vi "Read Waveform.vi"(0 "VISA resource name":refnum<visa-resource-name>, 5 "Trace Number (0: Scope Trace or Record)":i32(ring) items=["Scope Trace or Record", "Trend Plot", "Persistence", "Reference Trace", "Spectrum"], 7 "Channel (1: Channel A)":i32(ring)=1 items=["Channel A"=1, "Channel B"=2, "Channel C"=5, "Channel D"=6], 11 "error in (no error)":errorcluster) -> (3 "Y Unit":string, 4 "VISA resource name out":refnum<visa-resource-name>, 6 "Waveform":cluster{dbl[], "Max Data":dbl[]}[](graph), 8 "Overload":dbl format="%#_4e", 10 "Underload":dbl format="%#_4e", 14 "X Unit":string, 15 "error out":errorcluster)   [LabVIEW 2014, in "Fluke 190 Series II.lvlib"]
doc: "Reads and returns the trace data of a waveform from the Scopemeter."
uses:
  Fluke 190 Series II.lvlib
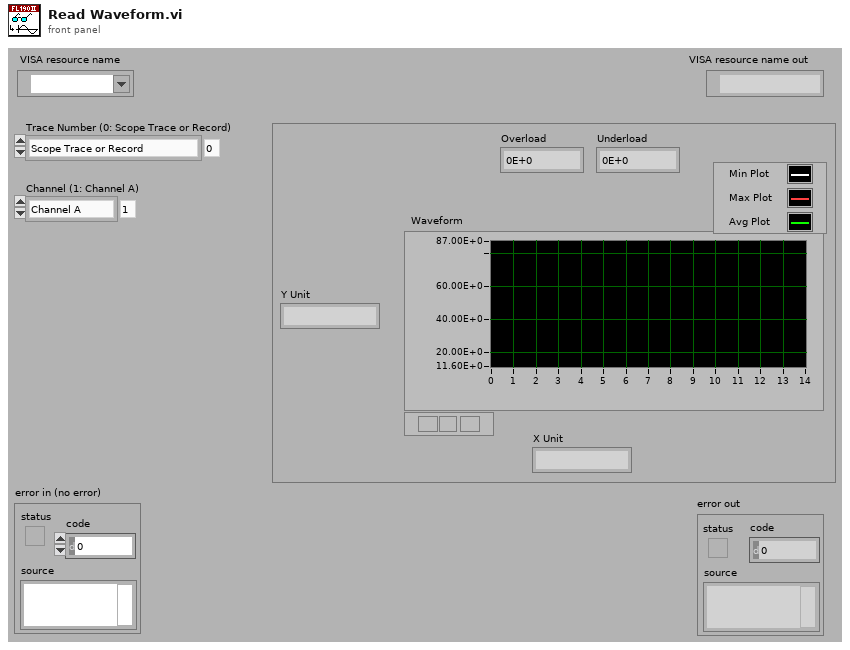
[diagram p1: front panel]
types:
  T1 = cluster{"Trace Result":u8, "Y Unit":u8, "X Unit ":u8, "Y Divisions":u16, "X Divisions":u16, "Y Scale":dbl, "X Scale":dbl, "Y Step":u8, "X Step":u8, "Y Offset":dbl, "X Offset":dbl, "Y Resolution":dbl, "X Resolution":dbl, "Y at 0":dbl, "X at 0":dbl, "Date Stamp":string, "Time Stamp":string}
  T2 = cluster{"Sample Format":i16, "Sample Pairing":u8, "Sample Byte Size":u8, "Overload":dbl, "Underload":dbl, "Invalid Samples":dbl, "Number of Samples":u16}
  T3 = cluster{"Min Data":dbl[], "Max Data":dbl[], "Avg Data":dbl[]}
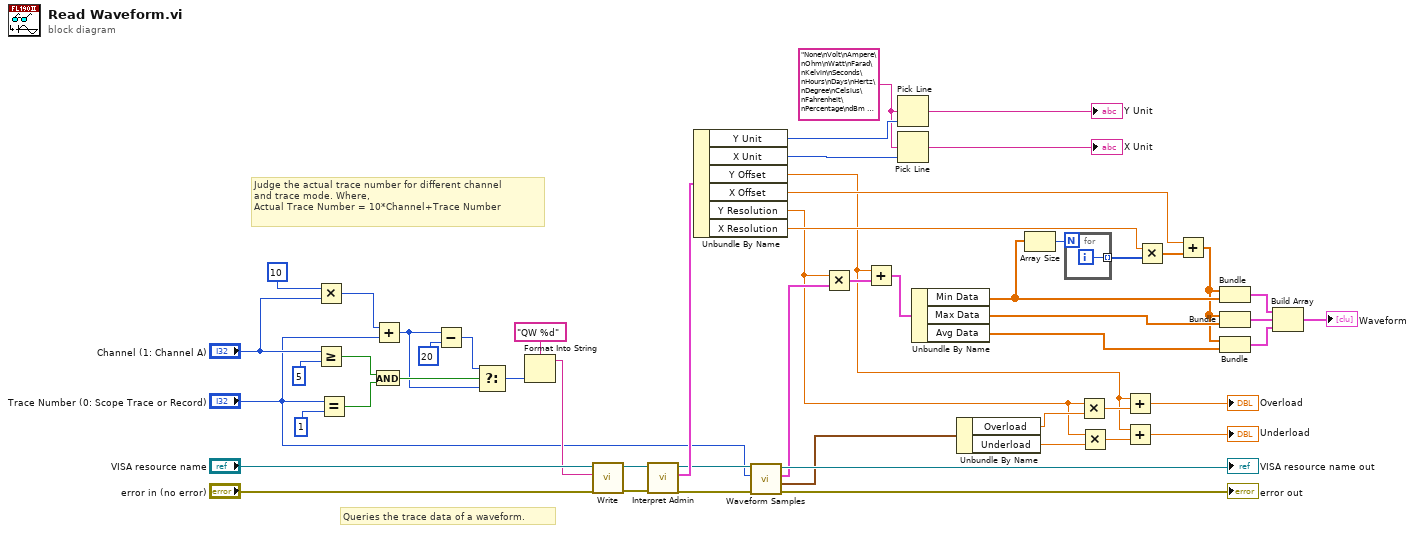
[diagram p0: block diagram]
diagram:
  w35 = "None\nVolt\nAmpere\nOhm\nWatt\nFarad\nKelvin\nSeconds\nHours\nDays\nHertz\nDegree\nCelsius\nFahrenheit\nPercentage\ndBm 50 Ohm\ndBm 600 Ohm\ndB Volts\ndB Ampere\ndB Watts\nVolt * Ampere Reactive\nVolt * Ampere" ("string (\"\")")
  # "Judge the actual trace number for different channel\nand trace mode. Where,\nActual Trace Number = 10*Channel+Trace Number"
  # "Queries the trace data of a waveform."
  n1 = Multiply(x=10, y="Channel (1: Channel A)") -> (x*y=w54:i32)
  n2 = Greater Or Equal?(x="Channel (1: Channel A)", y=5) -> (x >= y?=w47:bool)
  n3 = Equal?(x="Trace Number (0: Scope Trace or Record)", y=1) -> (x = y?=w49:bool)
  n4 = And(x=w47, y=w49) -> (x .and. y?=w46:bool)
  n5 = Add(x=w54, y="Trace Number (0: Scope Trace or Record)") -> (x+y=w41:i32)
  n6 = Subtract(x=w41, y=20) -> (x-y=w42:i32)
  n7 = Select(t=w42, s=w46, f=w41) -> (s? t:f=w22:i32)
  n8 = Format Into String(format string="QW %d", w22) -> (resulting string=w38:string)  [unwired: 2 in, 1 out]
  n9 = call "Write.vi"("error in (no error)"="error in (no error)", "Write Buffer"=w38, "VISA resource name"="VISA resource name") -> ("error out"=w39:errorcluster, "VISA resource name out"=w40:refnum<visa-resource-name>)  [unwired: 7 out]
  n10 = call "Interpret Admin.vi"("error in (no error)"=w39, "VISA resource name"=w40) -> ("error out"=w23:errorcluster, "Trace Admin"=w37:T1, "VISA resource name out"=w24:refnum<visa-resource-name>)  [unwired: 7 out]
  n11 = Unbundle By Name(w37) -> ("Y Unit"=w36:u8, "X Unit"=w34:u8, "Y Offset"=w10:dbl, "X Offset"=w12:dbl, "Y Resolution"=w11:dbl, "X Resolution"=w14:dbl)
  n12 = call "Waveform Samples.vi"("error in (no error)"=w23, "Trace Number (0: Scope Trace or Record)"="Trace Number (0: Scope Trace or Record)", "VISA resource name"=w24) -> ("error out"=→"error out":errorcluster, "Waveform Sample Information"=w19:T2, "Waveform Amplitude"=w18:T3, "VISA resource name out"=→"VISA resource name out":refnum<visa-resource-name>)  [unwired: 5 out]
  n13 = Multiply(x=w11, y=w18) -> (x*y=w17:T3)
  n14 = Add(x=w10, y=w17) -> (x+y=w16:T3)
  n15 = Pick Line(multi-line string=w35, line index=w36) -> (output string=→"Y Unit":string)  [unwired: 1 out]
  n16 = Pick Line(multi-line string=w35, line index=w34) -> (output string=→"X Unit":string)  [unwired: 1 out]
  n17 = Unbundle By Name(w16) -> ("Min Data"=w8:dbl[], "Max Data"=w7:dbl[], "Avg Data"=w2:dbl[])
  n18 = Unbundle By Name(w19) -> ("Overload"=w25:dbl, "Underload"=w31:dbl)
  n19 = Array Size(array=w8) -> (size(s)=w26:i32)
  n20 = for {
    N: w26 -> [_]
    tunnel: [w55] -> w15 mode=indexing
    i -> [w55]
  }
  n21 = Multiply(x=w11, y=w25) -> (x*y=w29:dbl)
  n22 = Multiply(x=w11, y=w31) -> (x*y=w30:dbl)
  n23 = Add(x=w10, y=w29) -> (x+y=→"Overload":dbl)
  n24 = Add(x=w10, y=w30) -> (x+y=→"Underload":dbl)
  n25 = Multiply(x=w14, y=w15) -> (x*y=w13:dbl[])
  n26 = Add(x=w12, y=w13) -> (x+y=w3:dbl[])
  n27 = Bundle(w3, "Min Data"=w8) -> (w6:cluster{dbl[], "Min Data":dbl[]})  [unwired: 1 out]
  n28 = Bundle(w3, "Max Data"=w7) -> (w5:cluster{dbl[], "Max Data":dbl[]})  [unwired: 1 out]
  n29 = Bundle(w3, "Avg Data"=w2) -> (w1:cluster{dbl[], "Avg Data":dbl[]})  [unwired: 1 out]
  n30 = Build Array(w6, w5, w1) -> (→"Waveform":cluster{dbl[], "Avg Data":dbl[]}[])
